vi "Global variable.vi"() -> ()   [LabVIEW 2020]
uses:
  Typedef/Mode.ctl
  Typedef/Schedule.ctl
  Typedef/Repeat.ctl
  Typedef/Action.ctl
  <vilib>/Utility/miscctls.llb/LVDateTimeRec.ctl
panel:
  in  "TCP ID":refnum<k5>
  in  "TCP Console":string
  in  "TCP MJPEG ID":refnum<k5>
  out "TCP connected":bool
  in  "Last update schedule":i32
  in  "Until schedule":T1[](array[typedef])
  out "Prev Mode":T2=enum."Realtime mode"
  in  "Schedules":T3[](array[typedef]) {"Action" items=["Turn off all", "Turn on all", "Fan on", "Fan off", "Light on", "Light off"]}
  in  "Global Ignore list":i32[](array[numeric])
  out "Mode":T2=enum."Realtime mode"
  in  "Global Error":errorcluster
  in  "Simulating":bool
  in  "Off delay":dbl=0.1
  in  "Off time":dbl
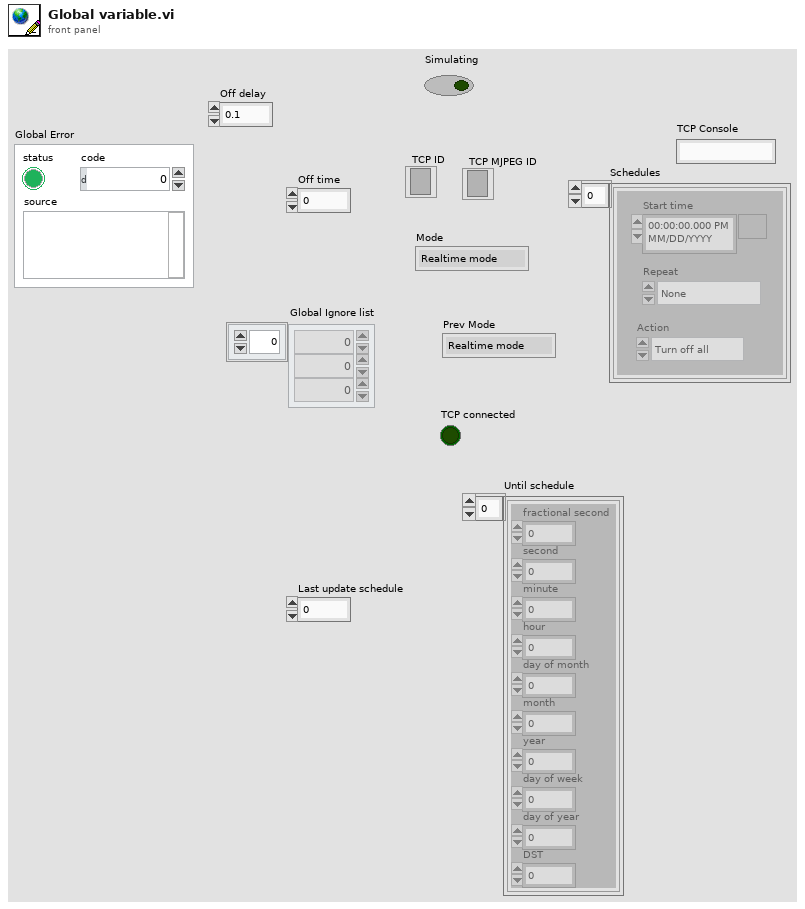
[diagram p1: front panel]
types:
  T1 = typedef "LVDateTimeRec.ctl" = cluster{"fractional second":dbl, "second":i32, "minute":i32, "hour":i32, "day of month":i32, "month":i32, "year":i32, "day of week":i32, "day of year":i32, "DST":i32}
  T2 = typedef "Mode.ctl" = enum16{"Schedule mode", "Manual mode", "Realtime mode", ""}
  T3 = typedef "Schedule.ctl" = cluster{"Start time":timestamp, "Repeat":T4, "Action":T5}
  T4 = typedef "Repeat.ctl" = enum16{"None", "Every hour", "Every day", "Every week", "Every month"}
  T5 = typedef "Action.ctl" = u16
diagram:
